vi "LaserCal-Init Meter (PT).vi"(0 "PM100":refnum<visa-resource-name>, 7 "Taverage":dbl, 11 "error in (no error)":errorcluster) -> (4 "PM100 thru":refnum<visa-resource-name>, 15 "error out":errorcluster)   [LabVIEW 2015]
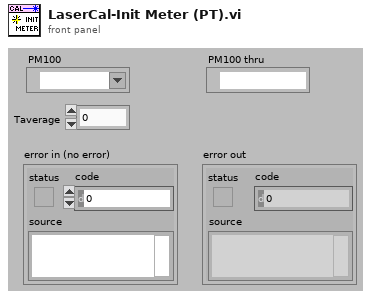
[diagram p1: front panel]
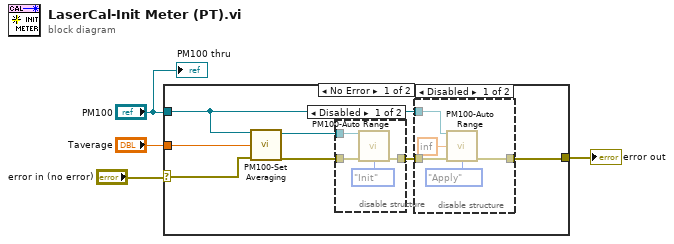
[diagram p0: block diagram]
diagram:
  n1 = case shown="No Error" "error in (no error)" {
    selector: "error in (no error)" -> [w6 w22]
    tunnel: [w5 w22] -> w3
    tunnel: "PM100" -> [w8 _]
    tunnel: "Taverage" -> [w11 _]
    frame No Error {
      n2 = call "PM100-Set Averaging.vi"("VISA in"=w8, "Average time (ms)"=w11, "error in (no error)"=w6) -> ("VISA out"=w10:refnum<visa-resource-name>, "error out"=w9:errorcluster)  [unwired: 11 in]
      n3 = disable-structure shown="Disabled" {
        disable-tunnel: w10 -> [w15 _]
        disable-tunnel: w9 -> [w14 w16]
        disable-tunnel: [w12 w16] -> w7
        frame Disabled {
          n4 = call "PM100-Auto Range.vi"("VISA in"=w15, "error in (no error)"=w14, "Action"=enum16{"Init", "Apply"}."Init") -> ("error out"=w12:errorcluster)  [unwired: 12 in]
        }
        frame Enabled {
        }
      }
      n5 = disable-structure shown="Disabled" {
        disable-tunnel: w8 -> [w20 _]
        disable-tunnel: w7 -> [w19 _]
        disable-tunnel: [w17 _] -> w5
        frame Disabled {
          n6 = call "PM100-Auto Range.vi"("VISA in"=w20, "Power (W)"=inf, "error in (no error)"=w19, "Action"=enum16{"Init", "Apply"}."Apply") -> ("error out"=w17:errorcluster)  [unwired: 11 in]
        }
        frame Enabled {
        }
      }
    }
    frame Error {
    }
  }
  "error out" <- w3
  "PM100 thru" <- "PM100"
